vi "PH_DeformableMirror.evt call Close.vi"(0 "i ref in":refnum<vi>, 1 "Object":string="N/A", 5 "error in (no error)":errorcluster) -> (14 "i ref out":refnum<vi>, 19 "error out":errorcluster)   [LabVIEW 2014, in "PH_DeformableMirror.lvlib"]
uses:
  PH_DeformableMirror.lvlib
  CSCore/BaseProcess/BaseProcess.lvlib
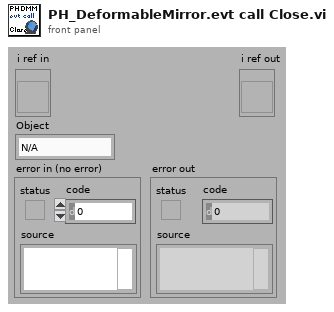
[diagram p1: front panel]
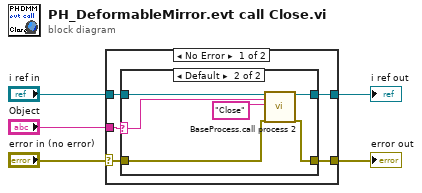
[diagram p0: block diagram]
diagram:
  n1 = case shown="No Error" "error in (no error)" {
    selector: "error in (no error)" -> [w7 w19]
    tunnel: "i ref in" -> [w10 w20]
    tunnel: [w9 w20] -> w4
    tunnel: [w8 w19] -> w3
    tunnel: "Object" -> [w6 _]
    frame No Error {
      n2 = case shown="Default" w6 {
        selector: w6 -> [_ w14]
        tunnel: w10 -> [w12 w18]
        tunnel: [w12 w17] -> w9
        tunnel: [w11 w16] -> w8
        tunnel: w7 -> [w11 w15]
        frame "", "N/A" {
        }
        frame Default {
          n3 = call "BaseProcess.call process 2.vi"("i ref in"=w18, "Object"=w14, "Selector"="Close", "error in (no error)"=w15) -> ("i ref out"=w17:refnum<vi>, "error out"=w16:errorcluster)  [unwired: 14 in]
        }
      }
    }
    frame Error {
    }
  }
  "error out" <- w3
  "i ref out" <- w4
